vi "pam system.vi"() -> ()   [LabVIEW 2019]
uses:
  <vilib>/addons/Control Design/_Model Conversions/NI_CD_Model Type.lvlib
  <vilib>/addons/Control Design/_Model Conversions/Model Type.llb/Model Conversion SubVI/cd_Convert State-Space to Transfer Function Model.vi
panel:
  in  "stop":bool
  in  "Pressure":dbl(slide) scale=0.0..1.0
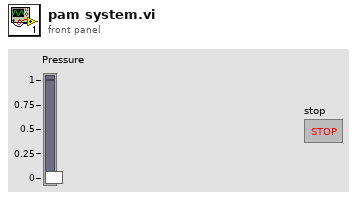
[diagram p1: front panel]
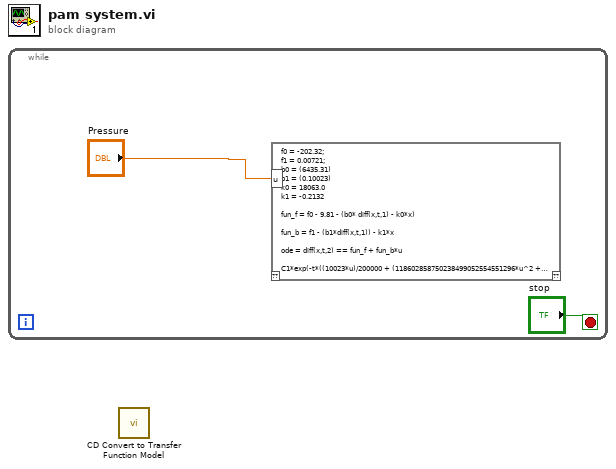
[diagram p0: block diagram]
diagram:
  n1 = while {
    stop <- "stop" stop-if-true
    n2 = mathscript code="f0 = -202.32;\nf1 = 0.00721;\nb0 = (6435.31)\nb1 = (0.10023)\nk0 = 18063.0\nk1 = -0.2132\n\nfun_f = f0 - 9.81 - (b0* diff(x,t,1) - k0*x)\n\nfun_b = f1 - (b1*diff(x,t,1)) - k1*x\n\node = diff(x,t,2) == fun_f + fun_b*u\n\nC1*exp(-t*((10023*u)/200000 + (118602858750238499052554551296*u^2 + 15239962586867914535757833830400000*u + 489773944810260575700212919566337890625)^(1/2)/6871947673600000 + 7075698173343171/2199023255552)) + C2*exp(-t*((10023*u)/200000 - (118602858750238499052554551296*u^2 + 15239962586867914535757833830400000*u + 489773944810260575700212919566337890625)^(1/2)/6871947673600000 + 7075698173343171/2199023255552)) - (721*u - 21213000)/(21320*u + 1806300000)"("u"="Pressure") -> ()  [unwired: 1 in, 1 out]
  }
  n3 = call-poly <vilib>:"CD Convert to Transfer Function Model.vi"() -> ()  [unwired: 10 in, 2 out]
